vi "Wykresy_skalujY_v2.vi"(7 "Wvm Ref in":refnum<vi>, 8 "error in (no error)":errorcluster, 11 "Data in":T1) -> (0 "error out":errorcluster, 2 "Przebiegi Wfm":waveform(dbl)[](array[waveform]), 4 "Kan i zakr":string[](array[string]))   [LabVIEW 2014]
doc: "Skaluje osie Y przebiegów przy uruchomieniu przetwarzania.\nOsie Enkowerowe - autoskala\nWszystkie przebiegi EN i AI na osobnych skalach\nPrzebiegi cyfrowe - skala nr 11 (12-sta skala) niewidoczna"
uses:
  Kontrolki/Przetwarzanie/Kanaly.ctl
  Kontrolki/GUI/Obsluga skal.ctl
  Zmienne/Zmienne globalne.vi
  Global variables.vi
panel:
  out "Chan name":string[](array[string])
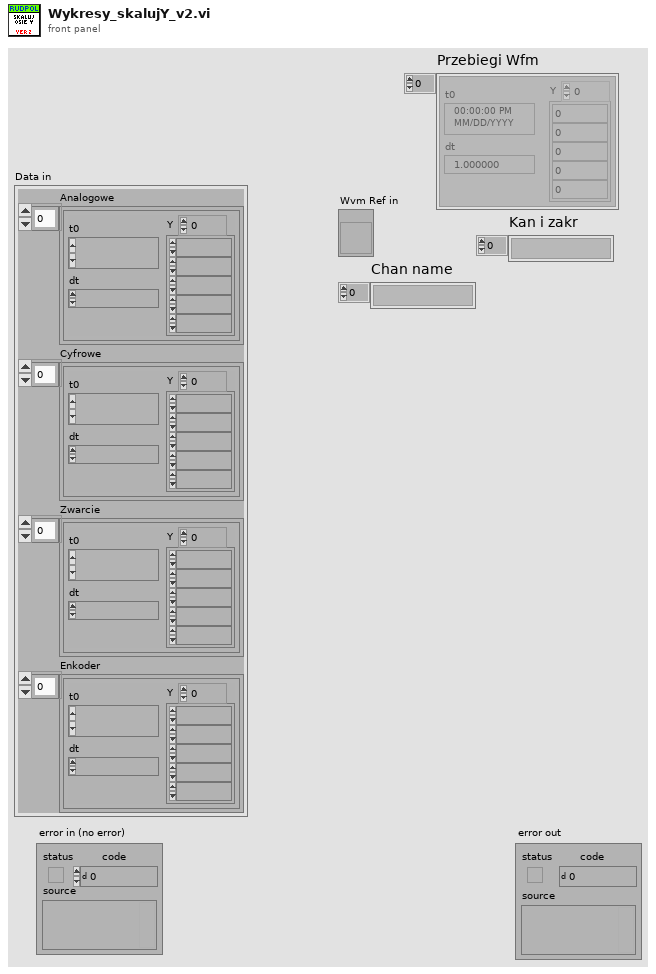
[diagram p1: front panel]
types:
  T1 = typedef "Kanaly.ctl" = cluster{"Analogowe":waveform(dbl)[], "Cyfrowe":waveform(dbl)[], "Zwarcie":waveform(dbl)[], "Enkoder":waveform(dbl)[]}
  T2 = typedef "Obsluga skal.ctl" = cluster{"Zakresy":dbl[], "skale":i32[], "Widoczna":bool[]}
  T3 = typedef "encoders data.ctl" = cluster{"S":dbl, "V":dbl, "a":dbl}
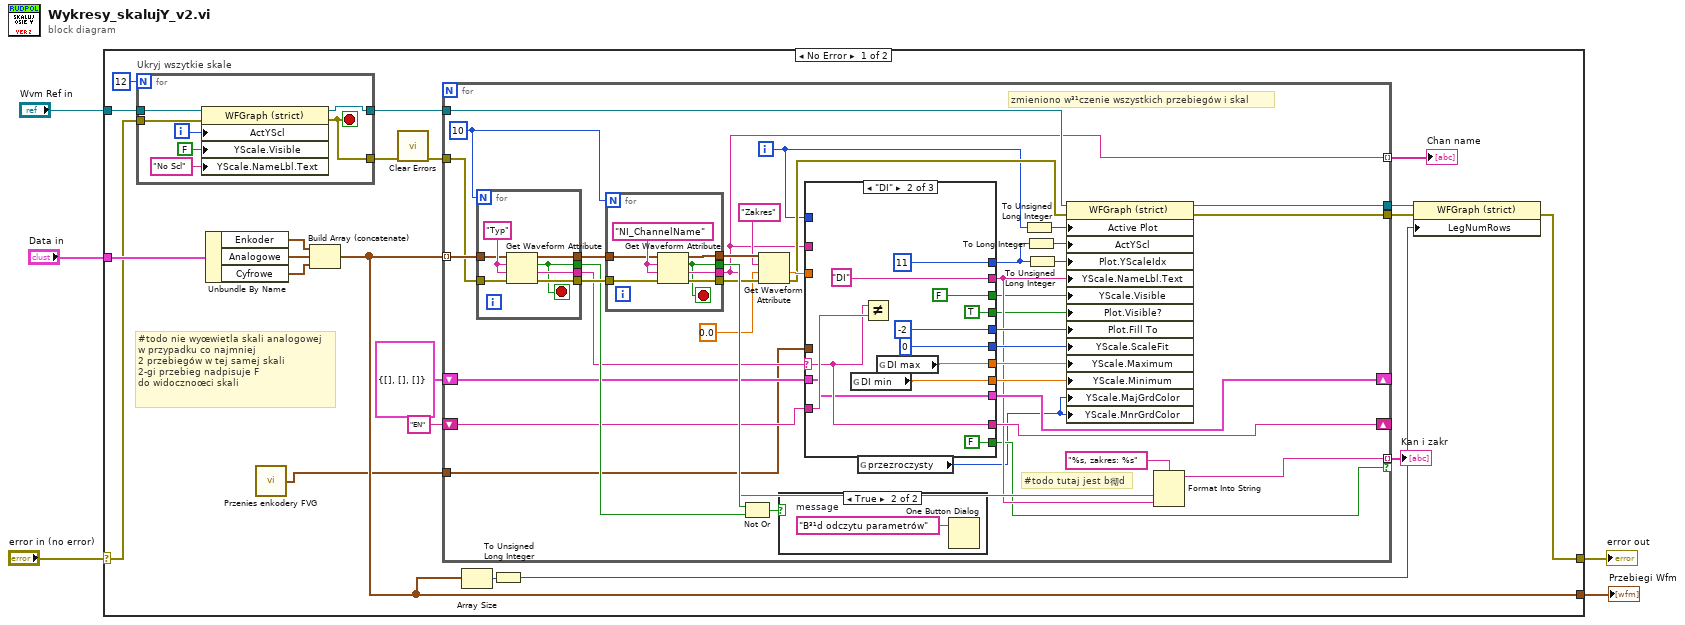
[diagram p0: block diagram]
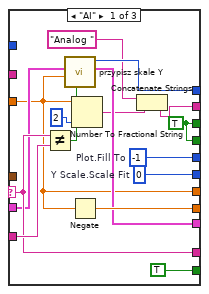
[diagram p2: hidden frame]
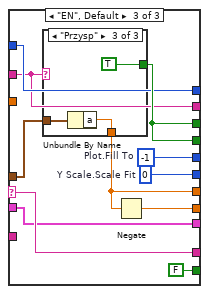
[diagram p3: hidden frame]
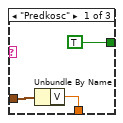
[diagram p4: hidden frame]
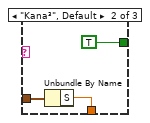
[diagram p5: hidden frame]
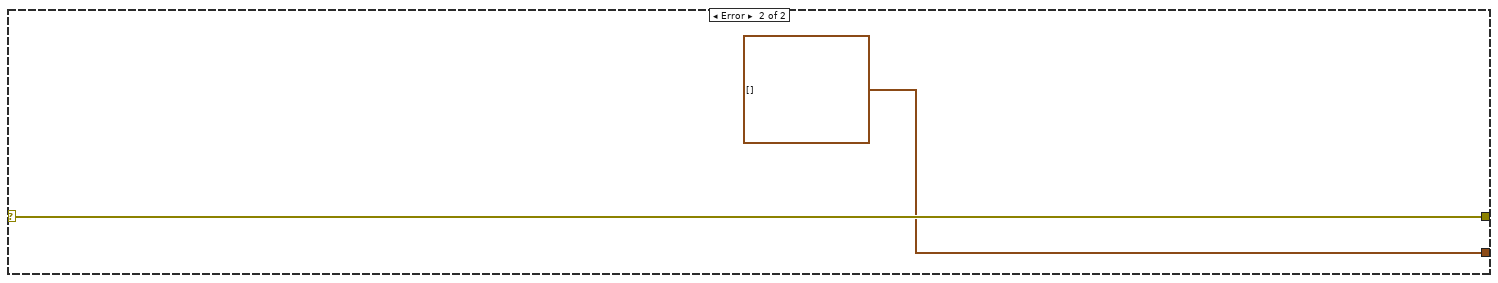
[diagram p7: hidden frame]
diagram:
  n1 = case shown="No Error" "error in (no error)" {
    selector: "error in (no error)" -> [w12 w138]
    tunnel: [w19 w138] -> w4
    tunnel: "Wvm Ref in" -> [w14 _]
    tunnel: "Data in" -> [w26 _]
    tunnel: [w17 waveform(dbl)[] []] -> w2
    frame No Error {
      # "#todo nie wyœwietla skali analogowej\nw przypadku co najmniej\n2 przebiegów w tej samej skali\n2-gi przebieg nadpisuje F\ndo widocznoœci skali"
      n2 = for "Ukryj wszytkie skale" {
        N: 12 -> [_]
        tunnel: w14 -> [w33]
        tunnel: [w30] -> w13
        tunnel: w12 -> [w29]
        tunnel: [w28] -> w10
        i -> [w31]
        stop <- w28 stop-if-true
        n3 = property class="WFGraph (strict)"(reference=w33, error in=w29, "ActYScl"=w31, "YScale.Visible"=FALSE ("Y Scale.Visible"), "YScale.NameLbl.Text"="No Scl" ("Y Scale.Name Label.Text")) -> (reference out=w30:refnum<vi>, error out=w28:errorcluster)
      }
      n4 = Unbundle By Name(w26) -> ("Enkoder"=w25:waveform(dbl)[], "Analogowe"=w24:waveform(dbl)[], "Cyfrowe"=w23:waveform(dbl)[])
      n5 = call "Przenies enkodery FVG.vi"() -> ("zakr out"=w6:T3)  [unwired: 10 in, 5 out]
      n6 = Build Array (concatenate)(w25, w24, w23) -> (w17:waveform(dbl)[])
      n7 = call <vilib>:"Clear Errors.vi"("error in (no error)"=w10) -> ("error out"=w11:errorcluster)  [unwired: 5 in, 1 out]
      n8 = for {
        tunnel: w17 -> [w71] mode=indexing
        tunnel: w13 -> [w60]
        shift-right: [w49] -> _
        shift-left: "EN" -> [w51]
        tunnel: [w35] -> w20
        tunnel: w11 -> [w50]
        tunnel: [w36] -> w21
        shift-right: [w45] -> _
        shift-left: T2 {"Zakresy"=[], "skale"=[], "Widoczna"=[]} ("Zakresy 2") -> [w46]
        tunnel: [w44] -> w8 mode=indexing
        tunnel: [w42] -> w7 mode=indexing if=w40
        tunnel: w6 -> [w39]
        i -> [w48]
        w70 = 10
        # "zmieniono w³¹czenie wszystkich przebiegów i skal"
        # "#todo tutaj jest b彻d"
        n9 = for {
          N: w70 -> [_]
          tunnel: [w135] -> w72
          tunnel: [w134] -> w73
          tunnel: w71 -> [w133]
          tunnel: [w132] -> w61
          tunnel: [w131] -> w67
          tunnel: w50 -> [w130]
          stop <- w131 stop-if-true
          w136 = "Typ"
          n10 = Get Waveform Attribute(4:w130, 5:w136, 6:w136, 7:w133) -> (0:w134:errorcluster, 1:w132:string, 2:w131:bool, 3:w135:waveform(dbl))
        }
        n11 = for {
          N: w70 -> [_]
          tunnel: w72 -> [w128]
          tunnel: w73 -> [w127]
          tunnel: [w126] -> w44
          tunnel: [w125] -> w65
          tunnel: [w124] -> w68
          tunnel: [w123] -> w66
          stop <- w124 stop-if-true
          w129 = "NI_ChannelName"
          n12 = Get Waveform Attribute(4:w127, 5:w129, 6:w129, 7:w128) -> (0:w125:errorcluster, 1:w126:string, 2:w124:bool, 3:w123:waveform(dbl))
        }
        n13 = Not Or(1:w67, 2:w68) -> (0:w69:bool)
        n14 = Get Waveform Attribute(4:w65, 5:0.0, 6:"Zakres", 7:w66) -> (0:w59:errorcluster, 1:w62:dbl)  [unwired: 2 out]
        n15 = case shown="True" w69 {
          frame False {
          }
          frame True {
            w122 = "B³¹d odczytu parametrów"  # message
            n16 = One Button Dialog(message=w122) -> ()  [unwired: 1 in, 1 out]
          }
        }
        n17 = case shown="\"DI\"" w61 {
          selector: w61 -> [w85 w97 w110]
          tunnel: [w89 i16 -2 ("Plot.Fill To") w112] -> w52
          tunnel: [w74 FALSE ("Y Scale.Visible") w109] -> w38
          tunnel: w62 -> [w81 _ _]
          tunnel: [w88 u8 0 ("Y Scale.Range:Maximum") w111] -> w53
          tunnel: [w81 w91 w103] -> w54
          tunnel: [w87 w92 w102] -> w55
          tunnel: w44 -> [_ _ w106]
          tunnel: [w85 w97 w110] -> w49
          tunnel: w51 -> [w86 w98 _]
          tunnel: [w74 TRUE ("Y Scale.Visible") w109] -> w37
          tunnel: w48 -> [_ _ w108]
          tunnel: [w83 11 w108] -> w47
          tunnel: w46 -> [w84 w95 w107]
          tunnel: [w82 w95 w107] -> w45
          tunnel: [w79 "DI" w106] -> w41
          tunnel: [TRUE FALSE FALSE] -> w40
          tunnel: w39 -> [_ _ w104]
          frame "AI" {
            w74 = TRUE ("Y Scale.Visible")
            w88 = u8 0  # Y Scale.Scale Fit
            w89 = i16 -1  # Plot.Fill To
            n18 = Not Equal?(x=w85, y=w86) -> (x != y?=w76:bool)
            n19 = call "przypisz skale Y.vi"("Visible in"=w76, "szukany zakres in"=w81, "Zakresy we"=w84) -> ("Zakresy wy"=w82:T2, "skala wy"=w83:i32)  [unwired: 5 in, 2 out]
            n20 = Negate(x=w81) -> (-x=w87:dbl)
            n21 = Number To Fractional String(number=w81, precision (6)=i16 2) -> (F-format string=w78:string)  [unwired: 2 in]
            n22 = Concatenate Strings("Analog " ("string"), w78) -> (w79:string)
          }
          frame "DI" {
            n23 = global read "Global variables.vi" "DI min"() -> (w92:dbl)
            n24 = Not Equal?(x=w97, y=w98) -> ()  [unwired: 1 out]
            n25 = global read "Global variables.vi" "DI max"() -> (w91:dbl)
          }
          frame "EN", Default {
            w111 = u8 0  # Y Scale.Scale Fit
            w112 = i16 -1  # Plot.Fill To
            n26 = case shown="\"Przysp\"" w106 {
              tunnel: [TRUE ("Y Scale.Visible") TRUE ("Y Scale.Visible") TRUE ("Y Scale.Visible")] -> w109
              tunnel: w104 -> [w114 w117 w120]
              tunnel: [w113 w116 w119] -> w103
              frame "Predkosc" {
                n27 = Unbundle By Name(w114) -> ("V"=w113:dbl)
              }
              frame "Kana³", Default {
                n28 = Unbundle By Name(w117) -> ("S"=w116:dbl)
              }
              frame "Przysp" {
                n29 = Unbundle By Name(w120) -> ("a"=w119:dbl)
              }
            }
            n30 = Negate(x=w103) -> (-x=w102:dbl)
          }
        }
        n31 = global read "Zmienne globalne.vi" "przezroczysty"() -> (w34:u32)
        n32 = To Unsigned Long Integer(number=w48) -> (unsigned 32bit integer=w58:u32)
        n33 = To Long Integer(number=w47) -> (32bit integer=w57:i32)
        n34 = To Unsigned Long Integer(number=w47) -> (unsigned 32bit integer=w56:u32)
        n35 = property class="WFGraph (strict)"(reference=w60, error in=w59, "Active Plot"=w58, "ActYScl"=w57, "Plot.YScaleIdx"=w56, "YScale.NameLbl.Text"=w41, "YScale.Visible"=w38, "Plot.Visible?"=w37, "Plot.Fill To"=w52, "YScale.ScaleFit"=w53, "YScale.Maximum"=w54, "YScale.Minimum"=w55, "YScale.MajGrdColor"=w34, "YScale.MnrGrdColor"=w34) -> (reference out=w35:refnum<vi>, error out=w36:errorcluster)
        n36 = Format Into String(format string="%s, zakres: %s", w44, w41) -> (resulting string=w42:string)  [unwired: 2 in, 1 out]
      }
      "Chan name" <- w8
      "Kan i zakr" <- w7
      n37 = Array Size(array=w17) -> (size(s)=w18:i32)
      n38 = To Unsigned Long Integer(number=w18) -> (unsigned 32bit integer=w16:u32)
      n39 = property on="Property Node" class="WFGraph (strict)"(reference=w20, error in=w21, "LegNumRows"=w16) -> (error out=w19:errorcluster)  [unwired: 1 out]
    }
    frame Error {
    }
  }
  "error out" <- w4
  "Przebiegi Wfm" <- w2
